vi "VFH-compare-R140_water_calib.vi"() -> ()   [LabVIEW 2020, in "VFH-VNA_File_Handler.lvlib"]
uses:
  VFH-VNA_File_Handler.lvlib
panel:
  out "Waveform Graph 2":dbl[](graph)
  out "Waveform Graph":dbl[](graph)
  out "error out 2":errorcluster
  out "error out":errorcluster
  out "Raw 2":T1(graph)
  in  "file path (dialog if empty) 2":path=path "C:/projects/UNI/VNA/MiniVNA/20240625-162312-Vann/Vann.txt"
  out "Raw":T1(graph)
  in  "file path (dialog if empty)":path=path "C:/projects/UNI/VNA/MiniVNA/20240625-162312-Vann/Vann.txt"
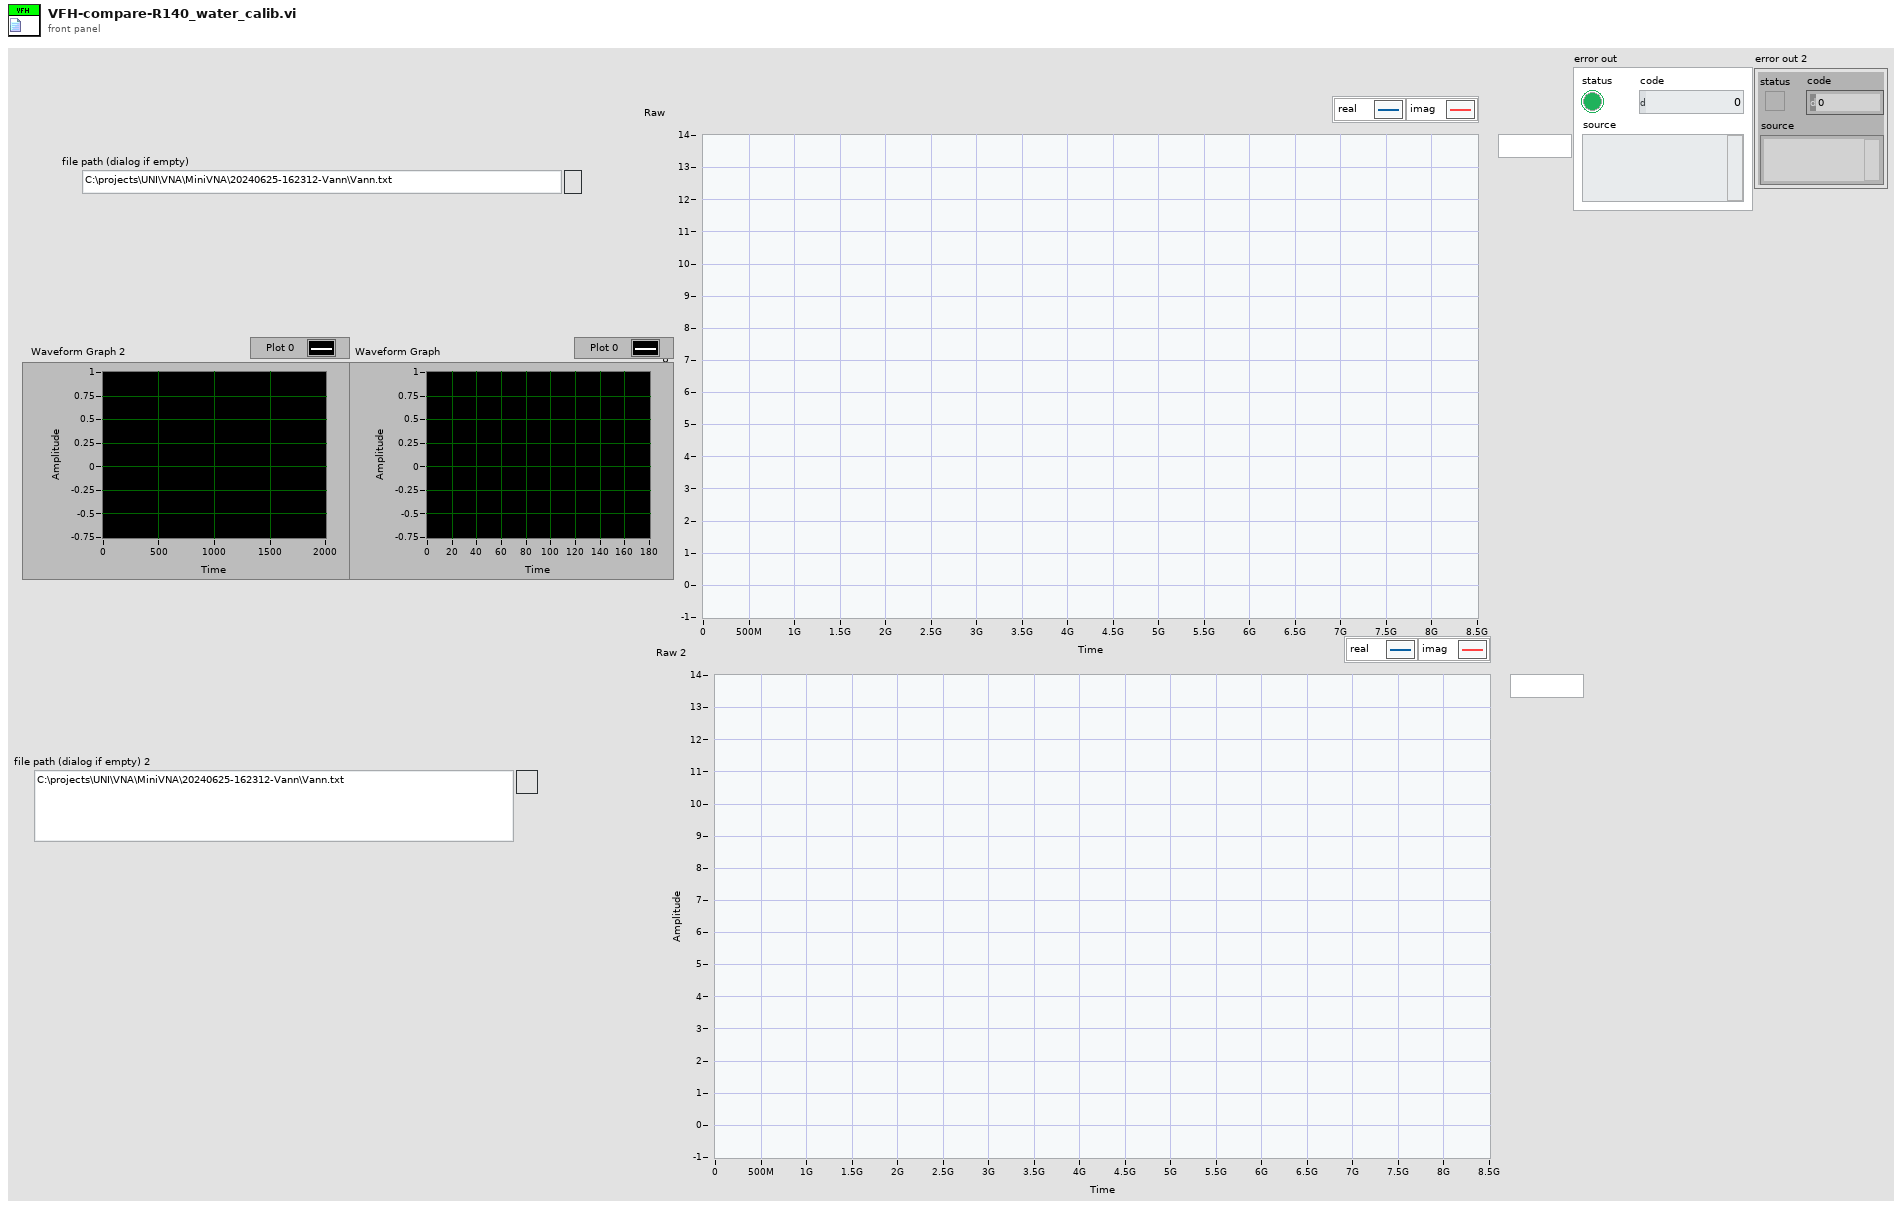
[diagram p1: front panel]
types:
  T1 = cluster{"Frequency":dbl[], "Reflection R":dbl[]}[]
  T2 = typedef "VFH-VNA_File_Handler.lvlib/VFH-file_cluster-R140.ctl" = cluster{"Frequency":dbl[], "Permativity'":dbl[], "Permativity''":dbl[], "Q [S/m]":dbl[], "Tan":dbl[], "Reflection R":dbl[], "Reflection I":dbl[]}
  T3 = typedef "VFH-VNA_File_Handler.lvlib/VFH-file_cluster-NanoVNA.ctl" = cluster{"Frequency":dbl[], "S11_Real":dbl[], "S11_Imag":dbl[], "S21_Real":dbl[], "S21_Imag":dbl[], "S12_Real":dbl[], "S12_Imag":dbl[], "S22_Real":dbl[], "S22_Imag":dbl[]}
  T4 = cluster{"Frequency":dbl[], "Reflection I":dbl[]}[]
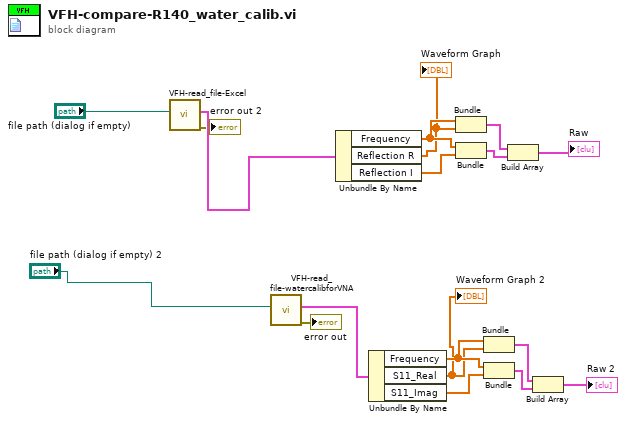
[diagram p0: block diagram]
diagram:
  n1 = call "VFH-read_file-Excel.vi"("file path (dialog if empty)"="file path (dialog if empty)") -> ("error out"=→"error out 2":errorcluster, "output cluster"=w13:T2)  [unwired: 9 in]
  n2 = call "VFH-read_file-watercalibforVNA.vi"("file path (dialog if empty)"="file path (dialog if empty) 2") -> ("error out"=→"error out":errorcluster, "output cluster"=w6:T3)  [unwired: 9 in]
  n3 = Unbundle By Name(w13) -> ("Frequency"=w3:dbl[], "Reflection R"=w2:dbl[], "Reflection I"=w18:dbl[])
  "Waveform Graph" <- w2
  n4 = Unbundle By Name(w6) -> ("Frequency"=w9:dbl[], "S11_Real"=w1:dbl[], "S11_Imag"=w8:dbl[])
  "Waveform Graph 2" <- w1
  n5 = Bundle("Frequency"=w3, "Reflection R"=w2) -> (w17:cluster{"Frequency":dbl[], "Reflection R":dbl[]})  [unwired: 1 in]
  n6 = Bundle("Frequency"=w3, "Reflection I"=w18) -> (w16:cluster{"Frequency":dbl[], "Reflection I":dbl[]})  [unwired: 1 in]
  n7 = Bundle("Frequency"=w9, "S11_Real"=w1) -> (w10:cluster{"Frequency":dbl[], "S11_Real":dbl[]})  [unwired: 1 in]
  n8 = Bundle("Frequency"=w9, "S11_Imag"=w8) -> (w11:cluster{"Frequency":dbl[], "S11_Imag":dbl[]})  [unwired: 1 in]
  n9 = Build Array(w17, w16) -> (→"Raw":T4)
  n10 = Build Array(w10, w11) -> (→"Raw 2":cluster{"Frequency":dbl[], "S11_Imag":dbl[]}[])
